vi "Write to Database.vi"(8 "error in":errorcluster, 9 "Array 2":T1(array[cluster]), 10 "Array":string[](array[string]), 11 "stripped path":path) -> (0 "error out":errorcluster, 2 "Table Name Out":string, 3 "appended path":path)   [LabVIEW 2019, in "flashcards.lvlib"]
uses:
  flashcards.lvlib
  <vilib>/addons/database/Auxilliary.llb/DB Tools DataTypes.ctl
  <vilib>/addons/database/Auxilliary.llb/DB Tools Column Info.ctl
  <vilib>/addons/database/Connection.llb/DB Tools Open Connec (String).vi
  <vilib>/addons/database/NI_Database_API.lvlib
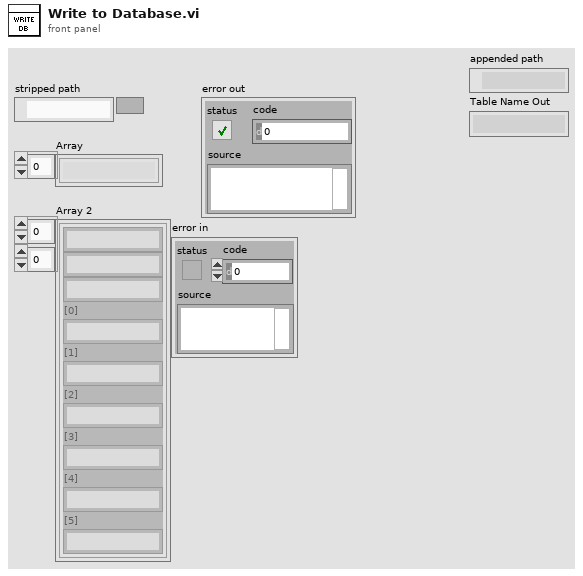
[diagram p1: front panel]
types:
  T1 = cluster{string, string, string, "[0]":string, "[1]":string, "[2]":string, "[3]":string, "[4]":string, "[5]":string}[][]
  T2 = typedef "NI_Database_API.lvlib/DB Tools Column Info.ctl" = cluster{"column name":string, "data type":T3, "size":i32, "allow null?":bool}
  T3 = typedef "NI_Database_API.lvlib/DB Tools DataTypes.ctl" = enum16{"String", "Long (I32)", "Single (SGL)", "Double (DBL)", "Date/Time", "Binary"}
  T4 = typedef "NI_Database_API.lvlib/Conn ObjectReference.ctl" = refnum<k1>
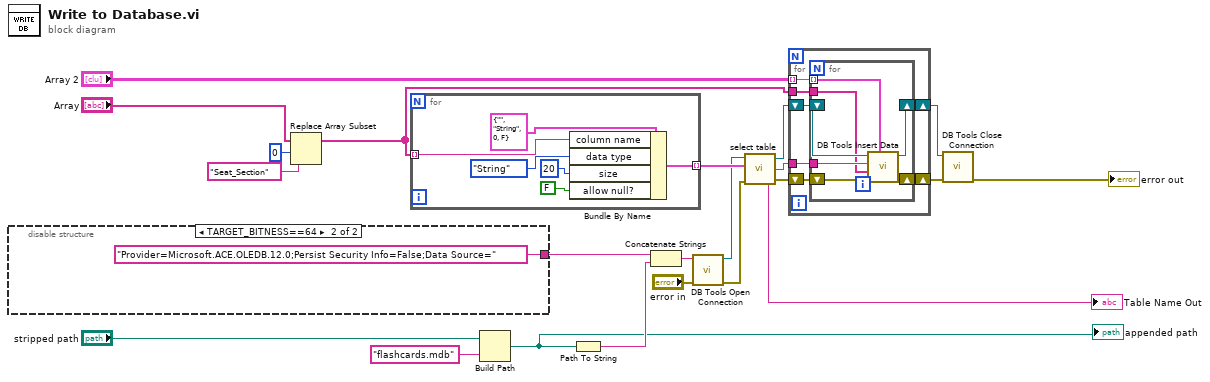
[diagram p0: block diagram]
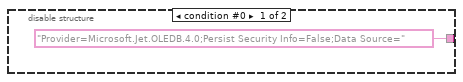
[diagram p2: hidden frame]
diagram:
  n1 = disable-structure shown="TARGET_BITNESS==64" {
    disable-tunnel: ["Provider=Microsoft.Jet.OLEDB.4.0;Persist Security Info=False;Data Source=" "Provider=Microsoft.ACE.OLEDB.12.0;Persist Security Info=False;Data Source="] -> w13
    frame condition #0 {
    }
    frame condition #1 (active) {
    }
  }
  n2 = Replace Array Subset(array="Array", new element="Seat_Section" ("new element/subarray"), index=0) -> (w3:string[])
  n3 = for {
    tunnel: [w29] -> w21 mode=indexing
    tunnel: w3 -> [w25] mode=indexing
    n4 = Bundle By Name(cluster=T2 {"column name"="", "data type"=enum."String", "size"=0, "allow null?"=FALSE} ("column information"), "column name"=w25, "data type"=DB_Tools_DataTypes."String", "size"=20, "allow null?"=FALSE) -> (w29:T2)
  }
  n5 = Build Path(base path="stripped path", name or relative path="flashcards.mdb") -> (appended path=w2:path)
  "appended path" <- w2
  n6 = Path To String(path=w2) -> (string=w12:string)
  n7 = Concatenate Strings(w13, w12) -> (w14:string)
  n8 = call-poly <vilib>:"DB Tools Open Connection.vi"("error in (no error)"="error in", "connection information"=w14) -> ("error out"=w11:errorcluster, "connection reference"=w9:T4)  [unwired: 6 in]
  n9 = call "select table.vi"("error in (no error)"=w11, "column information"=w21, "connection reference"=w9) -> ("error out"=w20:errorcluster, "Table Name Out"=w19:string, "connection reference out"=w15:T4)  [unwired: 1 in]
  "Table Name Out" <- w19
  n10 = for {
    shift-right: [w35] -> w16
    shift-left: w15 -> [w36]
    tunnel: "Array 2" -> [w33] mode=indexing
    tunnel: w19 -> [w32]
    tunnel: w3 -> [w31]
    shift-right: [w34] -> w17
    shift-left: w20 -> [w30]
    n11 = for {
      tunnel: w33 -> [w40] mode=indexing
      tunnel: w32 -> [w39]
      tunnel: w31 -> [w38]
      shift-right: [w42] -> w35
      shift-left: w36 -> [w43]
      shift-right: [w41] -> w34
      shift-left: w30 -> [w37]
      n12 = call <vilib>:"DB Tools Insert Data.vi"("data"=w40, "error in (no error)"=w37, "columns"=w38, "table"=w39, "connection reference"=w43) -> ("error out"=w41:errorcluster, "connection reference out"=w42:T4)  [unwired: 5 in]
    }
  }
  n13 = call <vilib>:"DB Tools Close Connection.vi"("error in (no error)"=w17, "connection reference"=w16) -> ("error out"=→"error out":errorcluster)  [unwired: 5 in]
